vi "_VNA_smith_reflection_GLOBALVARIABLES.vi"() -> ()   [LabVIEW 2013]
panel:
  out "Amplitude Background":cluster{dbl[], dbl[]}[](graph)
  out "Amplitude":cluster{dbl[], dbl[]}[](graph)
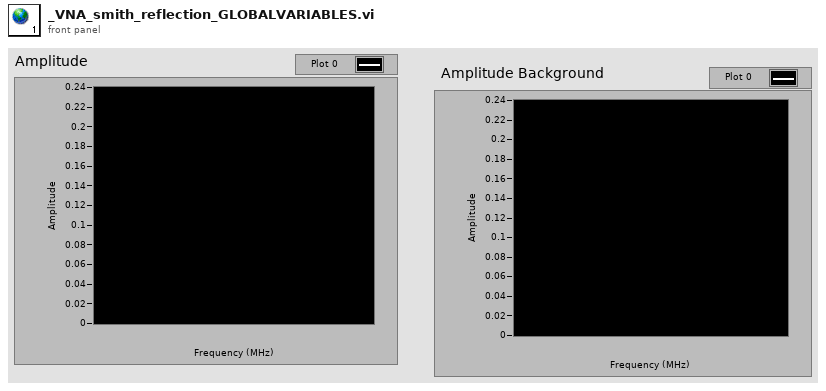
[diagram p1: front panel]
diagram:
